vi "Default File Name.vi"(8 "error in (no error)":errorcluster) -> (0 "error out":errorcluster, 3 "Default File Name":string)   [LabVIEW 2020, in "RxnRover.lvlib" / "User Preferences File.lvclass"]
doc: "Gets the default Rxn Rover user preferences file name based on the current operating system. The operating system name is read from OS.Name on a Application property node."
uses:
  User Preferences File.lvclass
  <vilib>/Utility/config.llb/Read Key (String).vi
  <vilib>/Utility/config.llb/NI_LVConfig.lvlib
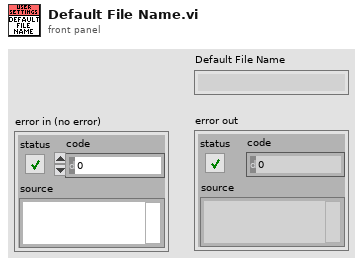
[diagram p1: front panel]
types:
  T1 = typedef "NI_LVConfig.lvlib/Config Data RefNum.ctl" = refnum<k1>
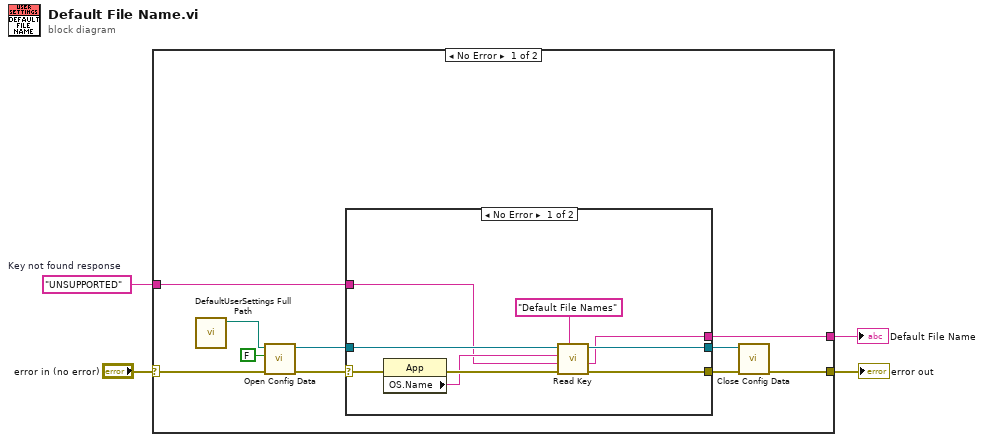
[diagram p0: block diagram]
diagram:
  w1 = "UNSUPPORTED"  # Key not found response
  n1 = case shown="No Error" "error in (no error)" {
    selector: "error in (no error)" -> [w14 w28]
    tunnel: [w10 w28] -> w3
    tunnel: [w9 w27] -> w2
    tunnel: w1 -> [w8 w27]
    frame No Error {
      n2 = call "DefaultUserSettings Full Path.vi"() -> ("DefaultUserSettings Full Path"=w6:path)  [unwired: 11 in]
      n3 = call <vilib>:"Open Config Data.vi"("error in (no error)"=w14, "create file if necessary (T)"=FALSE, "configuration file path"=w6) -> ("error out"=w5:errorcluster, "refnum"=w13:T1)  [unwired: 6 in, 1 out]
      n4 = case shown="No Error" w5 {
        selector: w5 -> [w15 w26]
        tunnel: w13 -> [w23 w25]
        tunnel: [w19 w26] -> w12
        tunnel: [w18 w25] -> w11
        tunnel: [w17 w24] -> w9
        tunnel: w8 -> [w16 w24]
        frame No Error {
          n5 = property class="App"(error in=w15) -> (error out=w22:errorcluster, "OS.Name"=w21:string)  [unwired: 1 in, 1 out]
          n6 = call-poly <vilib>:"Read Key.vi"("section"="Default File Names", "error in (no error)"=w22, "default value"=w16, "key"=w21, "refnum"=w23) -> ("error out"=w19:errorcluster, "value"=w17:string, "refnum out"=w18:T1)  [unwired: 3 in, 1 out]
        }
        frame Error {
        }
      }
      n7 = call <vilib>:"Close Config Data.vi"("error in (no error)"=w12, "refnum"=w11) -> ("error out"=w10:errorcluster)  [unwired: 8 in, 1 out]
    }
    frame Error {
    }
  }
  "error out" <- w3
  "Default File Name" <- w2
